vi "SMO.UI.GetPublicEvents.vi"(8 "error in (no error)":errorcluster, 11 "SMO.UI":refnum<class "SMO.UI.lvclass">) -> (0 "error out":errorcluster, 2 "SMO.UI Public Events":T1, 3 "SMO.UI out":refnum<class "SMO.UI.lvclass">)   [LabVIEW 2013, in "SMO.UI.lvclass"]
uses:
  SMO.UI.lvclass
  Typedefs/PublicEvents--Cluster.ctl
  SMO.UI.lvclass/SMO.UI.ctl
panel:
  # "For instructions on how to use the JKI State Machine Objects, examples and video tutorials, visit:\nhttp://jki.net/state-machine-objects/\n\nJKI State Machine Objects™\nhttp://jki.net/state-machine-objects/\nCopyright (C) 2005-2015, JKI <info@jki.net>\nALL RIGHTS RESERVED"
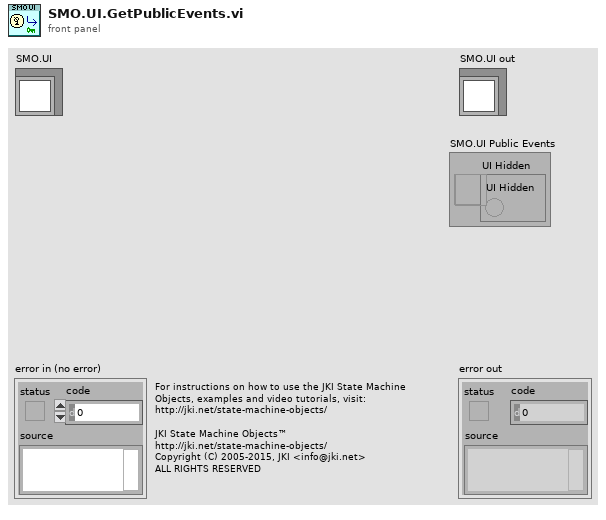
[diagram p1: front panel]
types:
  T1 = typedef "SMO.UI.lvclass/PublicEvents--Cluster.ctl" = cluster{"UI Hidden":refnum<user-event>}
  T2 = typedef "SMO.UI.lvclass/PrivateData--Ref.ctl" = refnum<data-value>
  T3 = typedef "SMO.UI.lvclass/PrivateData--Cluster.ctl" = cluster{"Public Events":T1, "Private Events":T4}
  T4 = typedef "SMO.UI.lvclass/PrivateEvents--Cluster.ctl" = cluster{"Show-Hide UI":refnum<user-event>}
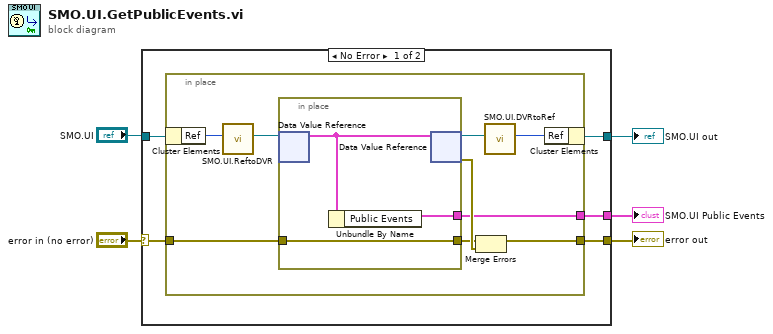
[diagram p0: block diagram]
diagram:
  n1 = case shown="No Error" "error in (no error)" {
    selector: "error in (no error)" -> [w9 w24]
    tunnel: [w8 w24] -> w2
    tunnel: [w7 w23] -> w4
    tunnel: "SMO.UI" -> [w10 w23]
    tunnel: [w6 _] -> w1
    frame No Error {
      n2 = in-place {
        in-place-border: w9 -> [w19]
        in-place-border: [w16] -> w8
        in-place-border: [w15] -> w6
        n3 = in-place-cluster #1(w10) -> ("Ref"=w14:u32)
        n4 = call "SMO.UI.ReftoDVR.vi"("Ref"=w14) -> ("Ref"=w13:T2)  [unwired: 10 in]
        n5 = in-place {
          in-place-border: w19 -> [w21]
          in-place-border: [w21] -> w17
          in-place-border: [w22] -> w15
          n6 = in-place-dvr #2(w13) -> (w20:T3)  [unwired: 1 out]
          n7 = Unbundle By Name(w20) -> ("Public Events"=w22:T1)
          n8 = in-place-dvr #2(w20) -> (w12:T2, w18:errorcluster)
        }
        n9 = Merge Errors(w17, w18) -> (w16:errorcluster)
        n10 = call "SMO.UI.DVRtoRef.vi"("Ref"=w12) -> ("Ref"=w11:u32)  [unwired: 10 in]
        n11 = in-place-cluster #1("Ref"=w11) -> (w7:refnum<class "SMO.UI.lvclass">)
      }
    }
    frame Error {
    }
  }
  "error out" <- w2
  "SMO.UI out" <- w4
  "SMO.UI Public Events" <- w1
